vi "peak comb -- interpolate - complex plane - V1.vi"(6 "peaks are known -- parameters":T1={"Def Gamma (kHz)"=0.0, "dV"=0.0, "time in Gamma (sec)"=0.0, "phi-star"=0.0, "all peaks (kHz)"=[564.0, 649.0, 987.0, 1133.0, 1214.0, 1585.0, 1763.0, 1823.0, 1880.0, 1899.0, 2032.0, 2138.0, 2221.0, 2270.0, 2350.0, 2456.0, 2580.0, 2634.0, 2831.0, 2960.0, 2965.0, 3131.0, 3328.0, 3469.0, 3553.0, 0.0, 3615.0, 3734.0, 0.0, 0.0, 0.0, 4236.0, 4300.0, 4331.0], "delta t (sec)"=0.0, "default step (Hz)"=0.0, "Max step (Hz)"=0.0, "all gamma (kHz)"=[564.0, 649.0, 987.0, 1133.0, 1214.0, 1585.0, 1763.0, 1823.0, 1880.0, 1899.0, 2032.0, 2138.0, 2221.0, 2270.0, 2350.0, 2456.0, 2580.0, 2634.0, 2831.0, 2960.0, 2965.0, 3131.0, 3328.0, 3469.0, 3553.0, 0.0, 3615.0, 3734.0, 0.0, 0.0, 0.0, 4236.0, 4300.0, 4331.0], "peaks OK"=FALSE, "gamma OK"=FALSE}, 9 "Gamma (kHz)":dbl=nan, 11 "freq (kHz)":dbl) -> (3 "delta-F (Hz)":dbl=-1.0)   [LabVIEW 2010]
uses:
  next chunk -- parameters.ctl
  Q - not nan -- real.vi
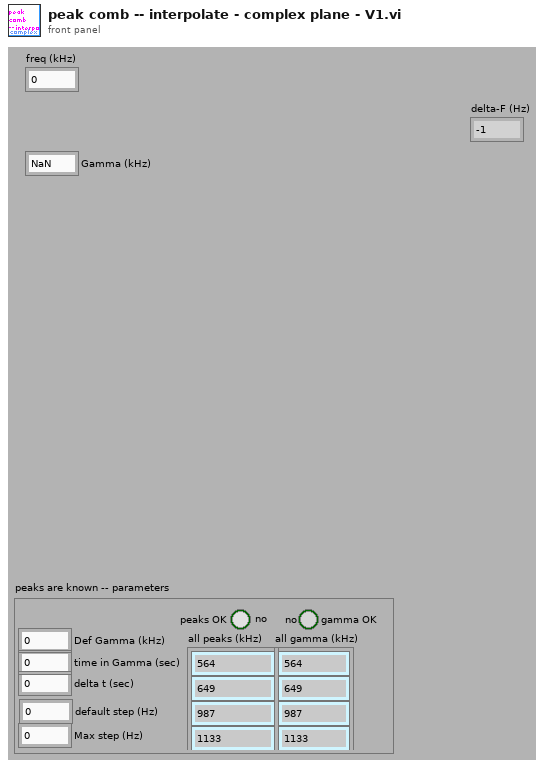
[diagram p1: front panel]
types:
  T1 = typedef "next chunk -- parameters.ctl" = cluster{"Def Gamma (kHz)":dbl, "dV":dbl, "time in Gamma (sec)":dbl, "phi-star":dbl, "all peaks (kHz)":dbl[], "delta t (sec)":dbl, "default step (Hz)":dbl, "Max step (Hz)":dbl, "all gamma (kHz)":dbl[], "peaks OK":bool, "gamma OK":bool}
  T2 = typedef "comparison control.ctl" = enum16{"not a number", "above", "in range", "below"}
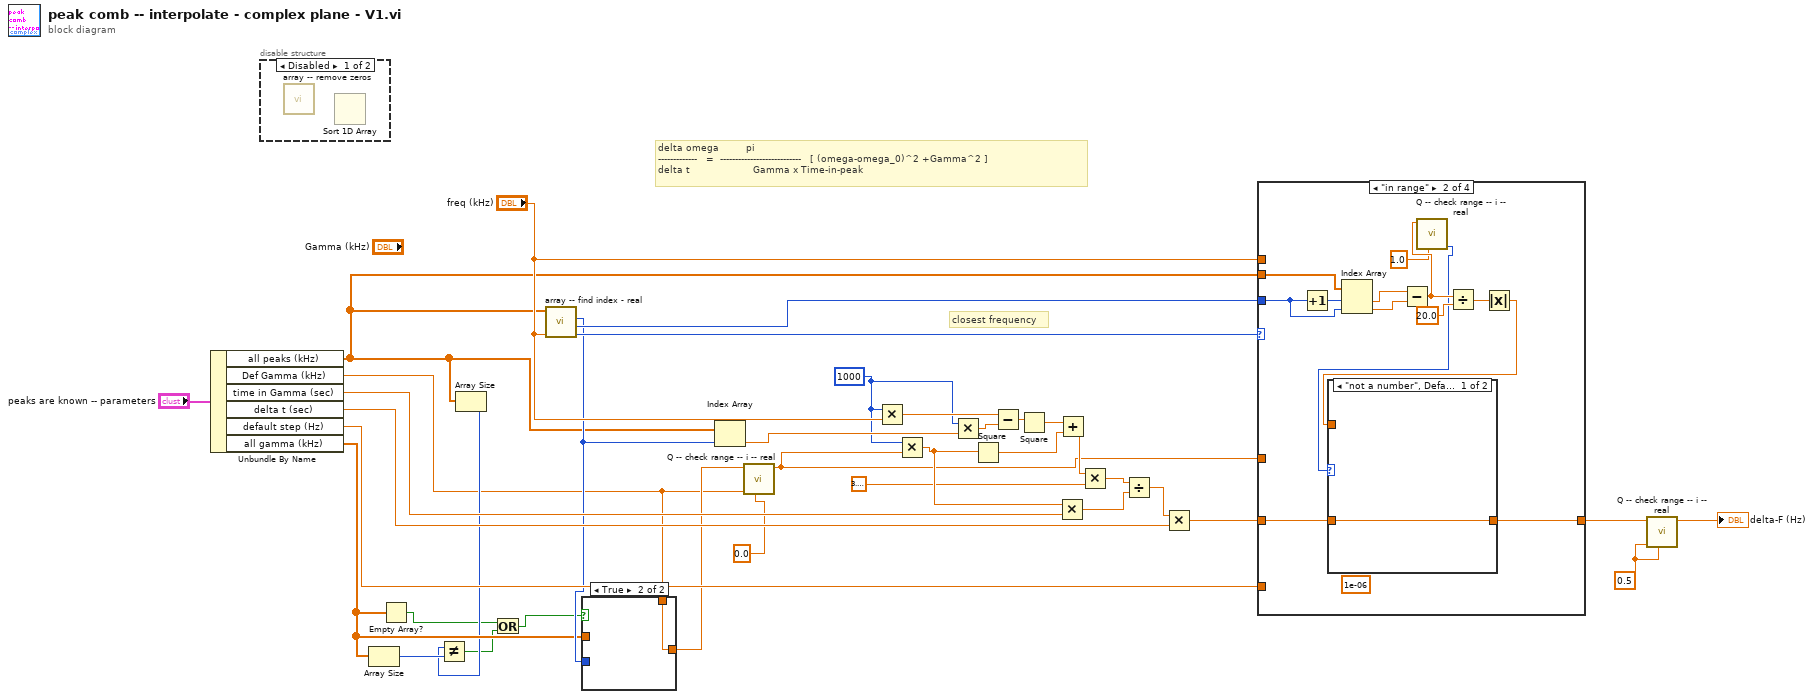
[diagram p0: block diagram]
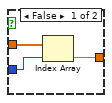
[diagram p2: hidden frame]
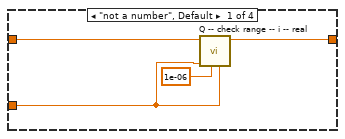
[diagram p4: hidden frame]
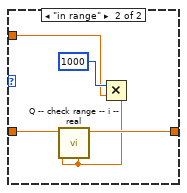
[diagram p5: hidden frame]
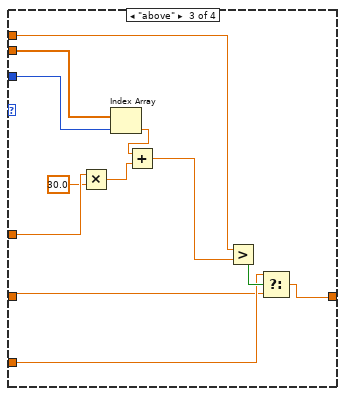
[diagram p6: hidden frame]
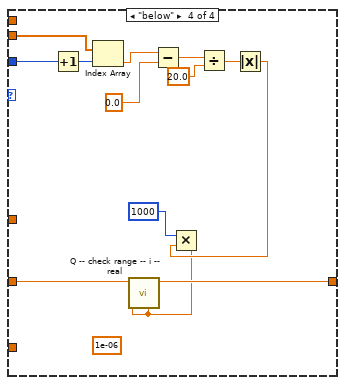
[diagram p7: hidden frame]
diagram:
  w1 = 0.5 ("default")
  w17 = 1000 ("dimension size")
  # "closest frequency"
  # "delta omega         pi\n-------------   =  ---------------------------   [ (omega-omega_0)^2 +Gamma^2 ] \ndelta t                     Gamma x Time-in-peak"
  n1 = Unbundle By Name("peaks are known -- parameters") -> ("all peaks (kHz)"=w11:dbl[], "Def Gamma (kHz)"=w4:dbl, "time in Gamma (sec)"=w35:dbl, "delta t (sec)"=w34:dbl, "default step (Hz)"=w27:dbl, "all gamma (kHz)"=w10:dbl[])
  n2 = disable-structure shown="Disabled" {
    frame Disabled {
      n3 = call "array -- remove zeros.vi"() -> ()  [unwired: 11 in, 1 out]
      n4 = Sort 1D Array() -> ()  [unwired: 1 in, 1 out]
    }
    frame Enabled {
    }
  }
  n5 = Array Size(array=w10) -> (size(s)=w9:i32)
  n6 = Empty Array?(array=w10) -> (empty?=w7:bool)
  n7 = Array Size(array=w11) -> (size(s)=w8:i32)
  n8 = Not Equal?(x=w8, y=w9) -> (x != y?=w6:bool)
  n9 = Or(x=w7, y=w6) -> (x .or. y?=w5:bool)
  n10 = call "array -- find index - real.vi"("number"="freq (kHz)", "temperatures"=w11) -> ("selector"=w31:T2, "left index"=w29:i32, "closest element index"=w14:i32)  [unwired: 6 in, 1 out]
  n11 = case shown="True" w5 {
    tunnel: w14 -> [w39 _]
    tunnel: [w38 w40] -> w13
    tunnel: w10 -> [w37 _]
    tunnel: w4 -> [_ w40]
    frame False {
      n12 = Index Array(array=w37, index=w39) -> (element=w38:dbl)
    }
    frame True {
    }
  }
  n13 = Index Array(array=w11, index=w14) -> (element=w33:dbl)
  n14 = call "Q -- check range -- i -- real.vi"("lower"=0.0, "default"=w4, "number"=w13) -> ("number in range"=w12:dbl)  [unwired: 6 in, 2 out]
  n15 = Multiply(x=w17, y="freq (kHz)") -> (x*y=w19:dbl)
  n16 = Multiply(x=w17, y=w12) -> (x*y=w16:dbl)
  n17 = Multiply(x=w17, y=w33) -> (x*y=w18:dbl)
  n18 = Square(x=w16) -> (x^2=w24:dbl)
  n19 = Subtract(x=w19, y=w18) -> (x-y=w26:dbl)
  n20 = Square(x=w26) -> (x^2=w25:dbl)
  n21 = Multiply(x=w16, y=w35) -> (x*y=w21:dbl)
  n22 = Add(x=w25, y=w24) -> (x+y=w23:dbl)
  n23 = Multiply(x=w23, y=3.141592653589793) -> (x*y=w22:dbl)
  n24 = Divide(x=w22, y=w21) -> (x/y=w20:dbl)
  n25 = Multiply(x=w20, y=w34) -> (x*y=w30:dbl)
  n26 = case shown="\"in range\"" w31 {
    tunnel: w30 -> [w43 w57 w64 w88]
    tunnel: w29 -> [_ w49 w74 w77]
    tunnel: w11 -> [_ w55 w75 w86]
    tunnel: "freq (kHz)" -> [_ _ w69 _]
    tunnel: [w41 w51 w65 w81] -> w3
    tunnel: w27 -> [w42 _ w66 _]
    tunnel: w12 -> [_ _ w72 _]
    frame "not a number", Default {
      n27 = call "Q -- check range -- i -- real.vi"("upper"=w42, "lower"=1e-06, "default"=w42, "number"=w43) -> ("number in range"=w41:dbl)  [unwired: 5 in, 2 out]
    }
    frame "in range" {
      (unwired) 1e-06 ("lower")
      n28 = Increment(x=w49) -> (x+1=w56:i32)
      n29 = Index Array(array=w55, index #1=w56, index #2=w49) -> (element #1=w54:dbl, element #2=w48:dbl)
      n30 = Subtract(x=w54, y=w48) -> (x-y=w47:dbl)
      n31 = call "Q -- check range -- i -- real.vi"("lower"=1.0, "number"=w47) -> ("selector"=w45:T2)  [unwired: 7 in, 2 out]
      n32 = Divide(x=w47, y=20.0) -> (x/y=w52:dbl)
      n33 = Absolute Value(x=w52) -> (abs(x)=w50:dbl)
      n34 = case shown="\"not a number\", Default" w45 {
        tunnel: w57 -> [w58 w63]
        tunnel: [w58 w62] -> w51
        tunnel: w50 -> [_ w60]
        frame "not a number", Default {
        }
        frame "in range" {
          n35 = Multiply(x=1000 ("dimension size"), y=w60) -> (x*y=w59:dbl)
          n36 = call "Q -- check range -- i -- real.vi"("upper"=w59, "default"=w59, "number"=w63) -> ("number in range"=w62:dbl)  [unwired: 6 in, 2 out]
        }
      }
    }
    frame "above" {
      n37 = Multiply(x=w72, y=30.0) -> (x*y=w70:dbl)
      n38 = Index Array(array=w75, index=w74) -> (element=w73:dbl)
      n39 = Add(x=w73, y=w70) -> (x+y=w68:dbl)
      n40 = Greater?(x=w69, y=w68) -> (0:w67:bool)
      n41 = Select(t=w66, s=w67, f=w64) -> (s? t:f=w65:dbl)
    }
    frame "below" {
      (unwired) 1e-06 ("lower")
      n42 = Increment(x=w77) -> (x+1=w87:i32)
      n43 = Index Array(array=w86, index=w87) -> (element=w85:dbl)
      n44 = Subtract(x=w85, y=0.0) -> (x-y=w84:dbl)
      n45 = Divide(x=w84, y=20.0) -> (x/y=w82:dbl)
      n46 = Absolute Value(x=w82) -> (abs(x)=w79:dbl)
      n47 = Multiply(x=1000 ("dimension size"), y=w79) -> (x*y=w78:dbl)
      n48 = call "Q -- check range -- i -- real.vi"("upper"=w78, "default"=w78, "number"=w88) -> ("number in range"=w81:dbl)  [unwired: 6 in, 2 out]
    }
  }
  n49 = call "Q -- check range -- i -- real.vi"("lower"=w1, "default"=w1, "number"=w3) -> ("number in range"=→"delta-F (Hz)":dbl)  [unwired: 6 in, 2 out]
